vi "CorrelImages (SubVI)v2.vi"(8 "last drift detected":i32, 9 "Correlate":u16(ring) items=["first Frame", "successive Frames"], 10 "Ref Array":dbl[][][](array[numeric]), 11 "New Image":dbl[][](array[numeric])) -> (2 "Y drift":i32, 3 "X drift":i32, 4 "Ref Array out":dbl[][][](array[numeric]), 5 "Queue Steps":i32=40)   [LabVIEW 2021]
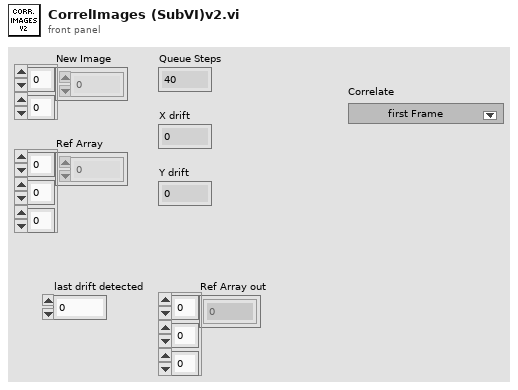
[diagram p1: front panel]
types:
  T1 = enum16{"nothing", "average", "8bit", "average/plane", "minimum", "plane", "average/stddev", "plane/average", "slope"}
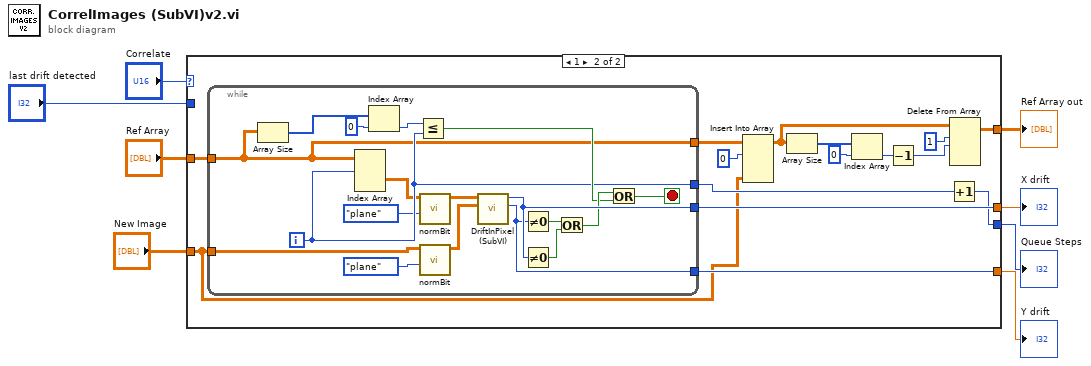
[diagram p0: block diagram]
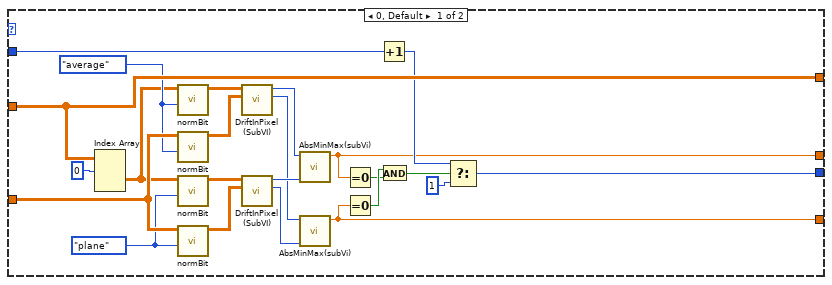
[diagram p2: hidden frame]
diagram:
  n1 = case shown="1" "Correlate" {
    tunnel: [w26 w32] -> w8
    tunnel: [w12 w45] -> w7
    tunnel: [w13 w44] -> w6
    tunnel: [w30 w37] -> w5
    tunnel: "New Image" -> [w19 w35]
    tunnel: "Ref Array" -> [w30 w33]
    tunnel: "last drift detected" -> [w24 _]
    frame 0, Default {
      w16 = T1."plane" ("method")
      w17 = T1."average" ("method")
      n2 = Index Array(array=w30, index (dim 0)=0 ("index (page)")) -> (element=w9:dbl[][])  [unwired: 2 in]
      n3 = call "normBit.vi"("method"=w17, "Rxy"=w9) -> ("Array"=w18:dbl[][])  [unwired: 8 in, 1 out]
      n4 = call "normBit.vi"("method"=w17, "Rxy"=w19) -> ("Array"=w22:dbl[][])  [unwired: 8 in, 1 out]
      n5 = call "normBit.vi"("method"=w16, "Rxy"=w9) -> ("Array"=w20:dbl[][])  [unwired: 8 in, 1 out]
      n6 = call "normBit.vi"("method"=w16, "Rxy"=w19) -> ("Array"=w21:dbl[][])  [unwired: 8 in, 1 out]
      n7 = call "DriftInPixel (SubVI).vi"("New image"=w22, "Ref image"=w18) -> ("Y drift"=w11:i32, "X drift"=w14:i32)  [unwired: 7 in, 1 out]
      n8 = call "DriftInPixel (SubVI).vi"("New image"=w21, "Ref image"=w20) -> ("Y drift"=w10:i32, "X drift"=w15:i32)  [unwired: 7 in, 1 out]
      n9 = call "AbsMinMax(subVi).vi"("y"=w15, "x"=w14) -> ("abs max"=w13:dbl)  [unwired: 8 in, 1 out]
      n10 = call "AbsMinMax(subVi).vi"("y"=w10, "x"=w11) -> ("abs max"=w12:dbl)  [unwired: 8 in, 1 out]
      n11 = Equal To 0?(x=w13) -> (x = 0?=w28:bool)
      n12 = Equal To 0?(x=w12) -> (x = 0?=w29:bool)
      n13 = Increment(x=w24) -> (x+1=w23:i32)
      n14 = And(x=w29, y=w28) -> (x .and. y?=w27:bool)
      n15 = Select(t=w23, s=w27, f=1) -> (s? t:f=w26:i32)
    }
    frame 1 {
      n16 = while {
        tunnel: w35 -> [w49]
        tunnel: w33 -> [w53]
        tunnel: [w62] -> w44
        tunnel: [w61] -> w45
        tunnel: [w57] -> w46
        tunnel: [w53] -> w34
        i -> [w57]
        stop <- w59 stop-if-true
        n17 = Array Size(array=w53) -> (size(s)=w56:i32[])
        n18 = Index Array(array=w53, index (dim 0)=w57) -> (element=w52:dbl[][])  [unwired: 2 in]
        n19 = Index Array(array=w56, index=0) -> (element=w54:i32)
        n20 = Less Or Equal?(x=w54, y=w57) -> (x <= y?=w58:bool)
        n21 = call "normBit.vi"("method"=T1."plane", "Rxy"=w52) -> ("Array"=w51:dbl[][])  [unwired: 8 in, 1 out]
        n22 = call "normBit.vi"("method"=T1."plane", "Rxy"=w49) -> ("Array"=w48:dbl[][])  [unwired: 8 in, 1 out]
        n23 = call "DriftInPixel (SubVI).vi"("New image"=w48, "Ref image"=w51) -> ("Y drift"=w61:i32, "X drift"=w62:i32)  [unwired: 7 in, 1 out]
        n24 = Not Equal To 0?(x=w61) -> (x != 0?=w64:bool)
        n25 = Not Equal To 0?(x=w62) -> (x != 0?=w63:bool)
        n26 = Or(x=w64, y=w63) -> (x .or. y?=w60:bool)
        n27 = Or(x=w60, y=w58) -> (x .or. y?=w59:bool)
      }
      n28 = Insert Into Array(array=w34, index (dim 0)=0 ("index (page)"), new element=w35) -> (w38:dbl[][][])  [unwired: 2 in]
      n29 = Array Size(array=w38) -> (size(s)=w39:i32[])
      n30 = Index Array(array=w39, index=0) -> (element=w41:i32)
      n31 = Decrement(x=w41) -> (x-1=w42:i32)
      n32 = Increment(x=w46) -> (x+1=w32:i32)
      n33 = Delete From Array(array=w38, length=1, index (dim 0)=w42) -> (array with subset deleted=w37:dbl[][][])  [unwired: 2 in, 1 out]
    }
  }
  "Queue Steps" <- w8
  "Y drift" <- w7
  "X drift" <- w6
  "Ref Array out" <- w5
